vi "_PC_NS_Signal_TimeSync.vi"(8 "error in (no error)":errorcluster) -> (0 "error out":errorcluster)   [LabVIEW 2018]
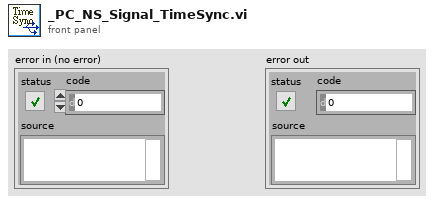
[diagram p1: front panel]
types:
  T1 = typedef "LVDateTimeRec.ctl" = cluster{"fractional second":dbl, "second":i32, "minute":i32, "hour":i32, "day of month":i32, "month":i32, "year":i32, "day of week":i32, "day of year":i32, "DST":i32}
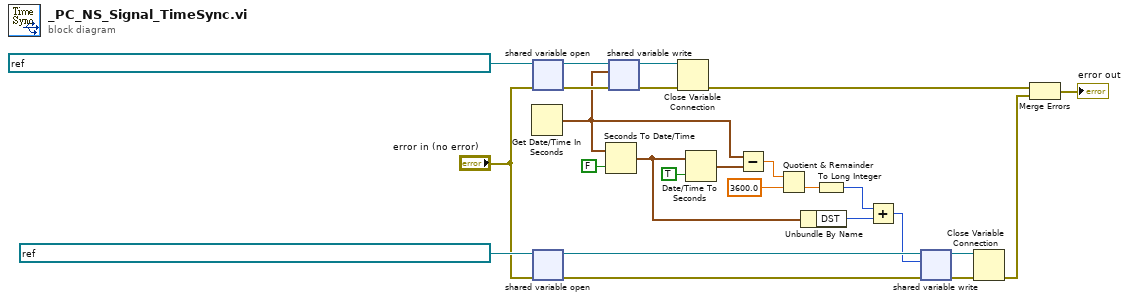
[diagram p0: block diagram]
diagram:
  n1 = Get Date/Time In Seconds() -> (seconds since 1Jan1904=w1:timestamp)
  n2 = shared-variable-open(refnum<k21> "ni.var.psp://NI-sbRIO/_RT_CtrlLoop_ResourcesMonitor_Variables/RT_timeupdate" ("shared variable refnum in"), "error in (no error)") -> (w25:refnum<k21>, w22:errorcluster)
  n3 = shared-variable-open(refnum<k21> "ni.var.psp://NI-sbRIO/_RT_CtrlLoop_ResourcesMonitor_Variables/RT TimeZone" ("shared variable refnum in"), "error in (no error)") -> (w7:refnum<k21>, w10:errorcluster)
  n4 = Seconds To Date/Time(time stamp (now)=w1, to UTC (F)=FALSE) -> (date time rec=w14:T1)
  n5 = shared-variable-write(w25, w22, w1) -> (w24:refnum<k21>, w23:errorcluster)
  n6 = Close Variable Connection(8:w23, 11:w24) -> (0:w4:errorcluster)
  n7 = Date/Time To Seconds(1:TRUE ("is UTC (F)"), 2:w14) -> (0:w15:timestamp)
  n8 = Subtract(x=w1, y=w15) -> (x-y=w16:dbl)
  n9 = Quotient & Remainder(x=w16, y=3600.0) -> (floor(x/y)=w18:dbl)  [unwired: 1 out]
  n10 = Unbundle By Name(w14) -> ("DST"=w12:i32)
  n11 = To Long Integer(number=w18) -> (32bit integer=w13:i32)
  n12 = Add(x=w13, y=w12) -> (x+y=w5:i32)
  n13 = shared-variable-write(w7, w10, w5) -> (w6:refnum<k21>, w11:errorcluster)
  n14 = Close Variable Connection(8:w11, 11:w6) -> (0:w3:errorcluster)
  n15 = Merge Errors(w4, w3) -> (→"error out":errorcluster)
